vi "Short Class Name to Variant.vi"(4 "KObject in":refnum<class "KObject.lvclass">) -> (1 "variant":variant)   [LabVIEW 2020, in "KObject.lvclass"]
uses:
  KObject.lvclass
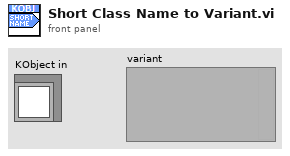
[diagram p1: front panel]
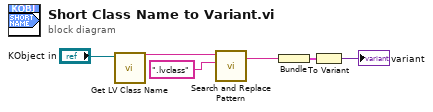
[diagram p0: block diagram]
diagram:
  n1 = call <vilib>:"Get LV Class Name.vi"("object"="KObject in") -> ("class name"=w5:string)  [unwired: 9 in, 1 out]
  n2 = call <vilib>:"Search and Replace Pattern.vi"("string"=w5, "regular expression (\"\")"=".lvclass" ("regular expression (\"\")")) -> ("result string"=w3:string)  [unwired: 3 in, 1 out]
  n3 = Bundle("result string"=w3) -> (w2:cluster{"result string":string})  [unwired: 1 in]
  n4 = To Variant(anything=w2) -> (Variant=→"variant":variant)
